vi "RunCameraPreview.vi"(8 "error in (no error)":errorcluster, 11 "CCD 3":refnum<vi>) -> (0 "error out":errorcluster)   [LabVIEW 2013]
uses:
  lib/System Files/user.lib/atmcd32d.llb/Error Code Enum typedef.ctl
  Variables/GetPicture.vi
  ccdChipPixels.vi
  StopGetPic.vi
panel:
  out "CCD 2":i32[][](graph)
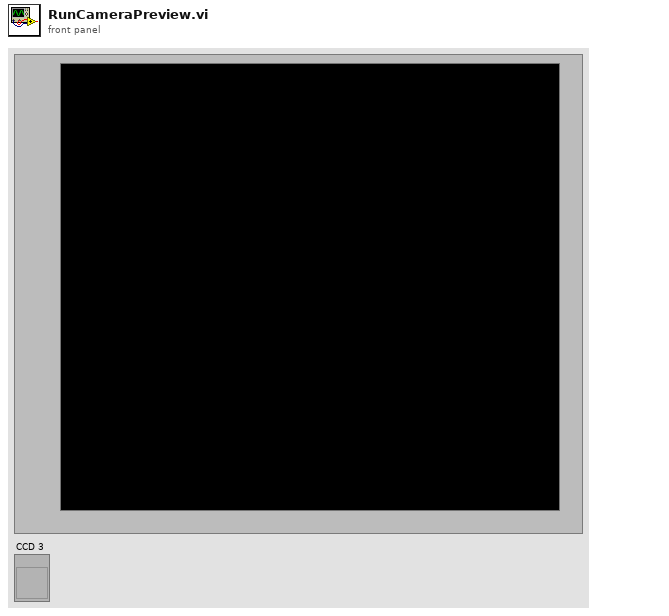
[diagram p1: front panel]
types:
  T1 = typedef "Error Code Enum typedef.ctl" = enum32{"N/A (0)", "DRV_ERROR_CODES", "DRV_SUCCESS", "DRV_VXDNOTINSTALLED", "DRV_ERROR_SCAN", "DRV_ERROR_CHECK_SUM", "DRV_ERROR_FILELOAD", "DRV_UNKNOWN_FUNC", "DRV_ERROR_VXD_INIT", "DRV_ERROR_ADDRESS", "DRV_ERROR_PAGELOCK", "DRV_ERROR_PAGEUNLOCK", "DRV_ERROR_BOARDTEST", "DRV_ERROR_ACK", "DRV_ERROR_UP_FIFO", "DRV_ERROR_PATTERN", "N/A (16)", "DRV_ACQUISITION_ERRORS", "DRV_ACQ_BUFFER", "DRV_ACQ_DOWNFIFO_FULL", "DRV_PROC_UNKONWN_INSTRUCTION", "DRV_ILLEGAL_OP_CODE", "DRV_KINETIC_TIME_NOT_MET", "DRV_ACCUM_TIME_NOT_MET", "DRV_NO_NEW_DATA", "N/A (25)", "DRV_SPOOLERROR", "N/A (27)", "N/A (28)", "N/A (29)", "N/A (30)", "N/A (31)", "N/A (32)", "DRV_TEMPERATURE_CODES", "DRV_TEMPERATURE_OFF", "DRV_TEMPERATURE_NOT_STABILIZED", "DRV_TEMPERATURE_STABILIZED", "DRV_TEMPERATURE_NOT_REACHED", "DRV_TEMPERATURE_OUT_RANGE", "DRV_TEMPERATURE_NOT_SUPPORTED", "DRV_TEMPERATURE_DRIFT", "N/A (41)", "N/A (42)", "N/A (43)", "N/A (44)", "N/A (45)", "N/A (46)", "N/A (47)", "N/A (48)", "DRV_GENERAL_ERRORS", "DRV_INVALID_AUX", "DRV_COF_NOTLOADED", "DRV_FPGAPROG", "DRV_FLEXERROR", "DRV_GPIBERROR", "N/A (55)", "N/A (56)", "N/A (57)", "N/A (58)", "N/A (59)", "N/A (60)", "N/A (61)", "N/A (62)", "N/A (63)", "DRV_DATATYPE", "DRV_DRIVER_ERRORS", "DRV_P1INVALID", "DRV_P2INVALID", "DRV_P3INVALID", "DRV_P4INVALID", "DRV_INIERROR", "DRV_COFERROR", "DRV_ACQUIRING", "DRV_IDLE", "DRV_TEMPCYCLE", "DRV_NOT_INITIALIZED", "DRV_P5INVALID", "DRV_P6INVALID", "DRV_INVALID_MODE", "DRV_INVALID_FILTER", "DRV_I2CERRORS", "DRV_I2CDEVNOTFOUND", "DRV_I2CTIMEOUT", "DRV_P7INVALID", "N/A (84)", "N/A (85)", "N/A (86)", "N/A (87)", "N/A (88)", "N/A (89)", "DRV_IOCERROR", "DRV_VRMVERSIONERROR"}
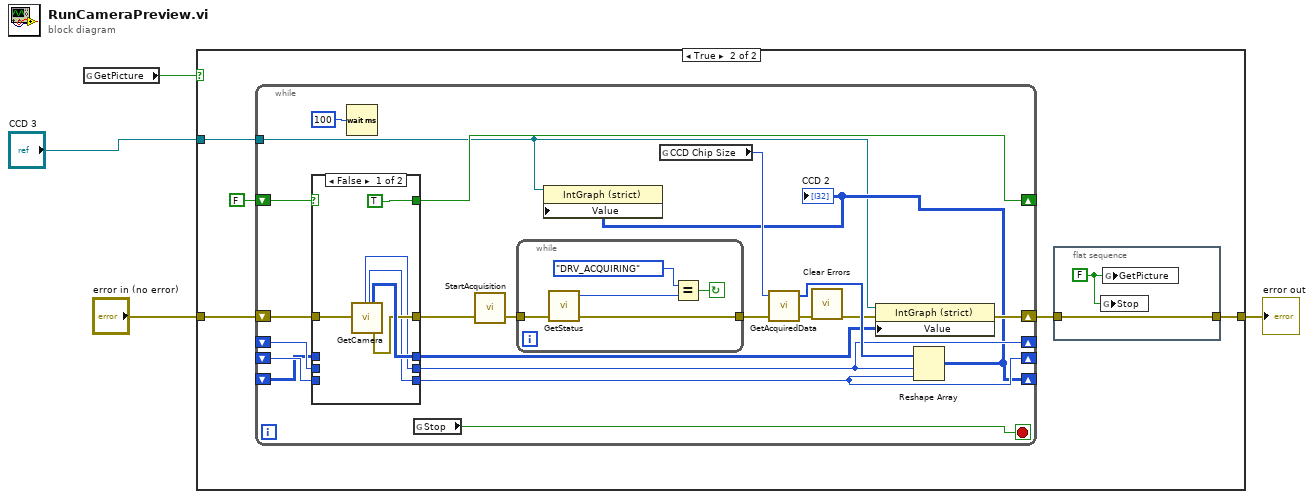
[diagram p0: block diagram]
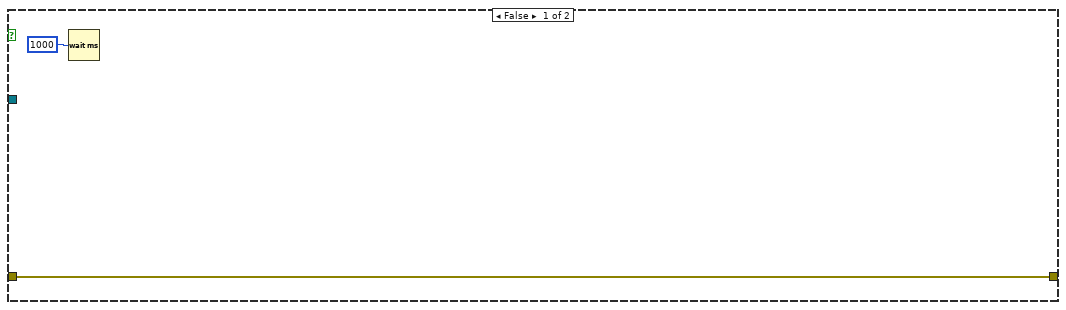
[diagram p2: hidden frame]
diagram:
  n1 = global read "GetPicture.vi" "GetPicture"() -> (w2:bool)
  n2 = case shown="True" w2 {
    tunnel: "error in (no error)" -> [w6 w10]
    tunnel: [w6 w9] -> w4
    tunnel: "CCD 3" -> [_ w7]
    frame False {
      n3 = Wait (ms)(milliseconds to wait=u32 1000) -> ()  [unwired: 1 out]
    }
    frame True {
      n4 = while {
        shift-right: [w19] -> w8
        shift-left: w10 -> [w32]
        shift-right: [w26] -> _
        shift-left: FALSE -> [w20]
        shift-right: [w24] -> _
        shift-left: _ -> [w23]
        shift-right: [w25] -> _
        shift-left: _ -> [w22]
        shift-right: [w13] -> _
        shift-left: _ -> [w21]
        tunnel: w7 -> [w12]
        stop <- w17 stop-if-true
        n5 = case shown="False" w20 {
          selector: w20 -> [_ w39]
          tunnel: w32 -> [w38 w43]
          tunnel: [w37 w40] -> w16
          tunnel: [w36 w43] -> w27
          tunnel: [TRUE w39] -> w26
          tunnel: [w34 w42] -> w24
          tunnel: [w33 w41] -> w25
          tunnel: w23 -> [_ w42]
          tunnel: w22 -> [_ w41]
          tunnel: w21 -> [_ w40]
          frame False {
            n6 = call "GetCamera.vi"("error out 2"=w38) -> ("CCD Chip horizontal end"=w34:i32, "CCD Chip Vertical end"=w33:i32, "array"=w37:i32[][], "error out"=w36:errorcluster)  [unwired: 20 in, 3 out]
          }
          frame True {
          }
        }
        n7 = Wait (ms)(milliseconds to wait=u32 100) -> ()  [unwired: 1 out]
        n8 = global read "StopGetPic.vi" "Stop"() -> (w17:bool)
        n9 = call "StartAcquisition.vi"("error in (no error)"=w27) -> ("error out"=w30:errorcluster)  [unwired: 1 in, 1 out]
        n10 = while {
          tunnel: w30 -> [w48]
          tunnel: [w47] -> w29
          stop <- w44 continue-if-true
          n11 = call "GetStatus.vi"("error in (no error)"=w48) -> ("error out"=w47:errorcluster, "status"=w45:T1)  [unwired: 2 in, 1 out]
          n12 = Equal?(x=Error_Code_Enum_typedef."DRV_ACQUIRING" ("status"), y=w45) -> (x = y?=w44:bool)
        }
        n13 = global read "ccdChipPixels.vi" "CCD Chip Size"() -> (w14:i32)
        n14 = call "GetAcquiredData.vi"("error in (no error)"=w29, "size"=w14) -> ("error out"=w28:errorcluster, "array"=w31:i32[])  [unwired: 1 in, 1 out]
        n15 = call <vilib>:"Clear Errors.vi"("error in (no error)"=w28) -> ("error out"=w15:errorcluster)  [unwired: 6 in]
        n16 = property on="Property Node" class="IntGraph (strict)"(reference=w12, error in=w15, "Value"=w16) -> (error out=w19:errorcluster)  [unwired: 1 out]
        n17 = Reshape Array(w31, w24, w25) -> (w13:i32[][])
        "CCD 2" <- w13
        n18 = property class="IntGraph (strict)"(reference=w12, "Value"=w13) -> ()  [unwired: 1 in, 2 out]
      }
      n19 = flat-sequence {
        tunnel: [w50] -> w9
        tunnel: w8 -> [w50]
        frame #0 {
          w49 = FALSE ("GetPicture")
          n20 = global write "StopGetPic.vi" "Stop"(w49) -> ()
          n21 = global write "GetPicture.vi" "GetPicture"(w49) -> ()
        }
      }
    }
  }
  "error out" <- w4
